vi "Denkovi_USB_4_8_RelayDemo.vi"() -> ()   [LabVIEW 2018]
panel:
  out "FT_Status":u32(ring) items=["FT_OK", "FT_INVALID_HANDLE", "FT_DEVICE_NOT_FOUND", "FT_DEVICE_NOT_OPENED", "FT_IO_ERROR", "FT_INSUFFICIENT_RESOURCES", "FT_INVALID_PARAMETER", "FT_INVALID_BAUD_RATE", "FT_DEVICE_NOT_OPENED_FOR_ERASE", "FT_DEVICE_NOT_OPENED_FOR_WRITE", "FT_FAILED_TO_WRITE_DEVICE", "FT_EEPROM_READ_FAILED", "FT_EEPROM_WRITE_FAILED", "FT_EEPROM_ERASE_FAILED", "FT_EEPROM_NOT_PRESENT", "FT_EEPROM_NOT_PROGRAMMED", "FT_INVALID_ARGS", "FT_NOT_SUPPORTED", "FT_OTHER_ERROR"]
  out "Device Description":string
  out "Pin States":T1
  in  "ALL ON/OFF":bool
  in  "DO7":bool
  in  "DO6":bool
  in  "DO5":bool
  in  "DO4":bool
  in  "DO3":bool
  in  "DO2":bool
  in  "DO1":bool
  in  "DO0":bool
  in  "Device Index":u32
  # "LabView demo example for USB 4/8 Relay Board by Denkovi\nDemonstrates how to read and write USB relay board I/O lines (relays). Uses the FTDI D2XX functions."
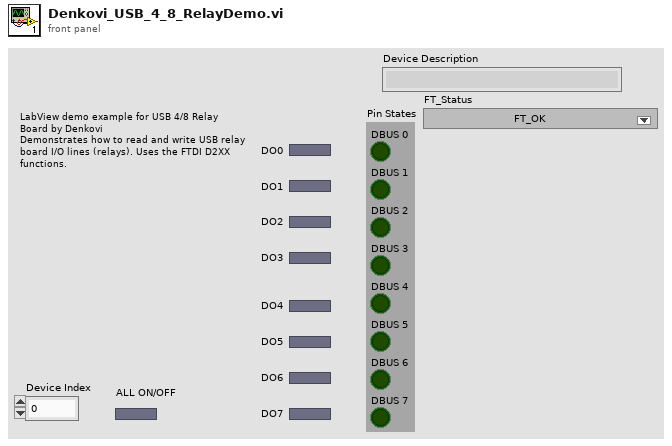
[diagram p1: front panel]
types:
  T1 = cluster{"DBUS 0":bool, "DBUS 1":bool, "DBUS 2":bool, "DBUS 3":bool, "DBUS 4":bool, "DBUS 5":bool, "DBUS 6":bool, "DBUS 7":bool}
  T2 = cluster{"Boolean array[0]":bool, "Boolean array[1]":bool, "Boolean array[2]":bool, "Boolean array[3]":bool, "Boolean array[4]":bool, "Boolean array[5]":bool, "Boolean array[6]":bool, "Boolean array[7]":bool}
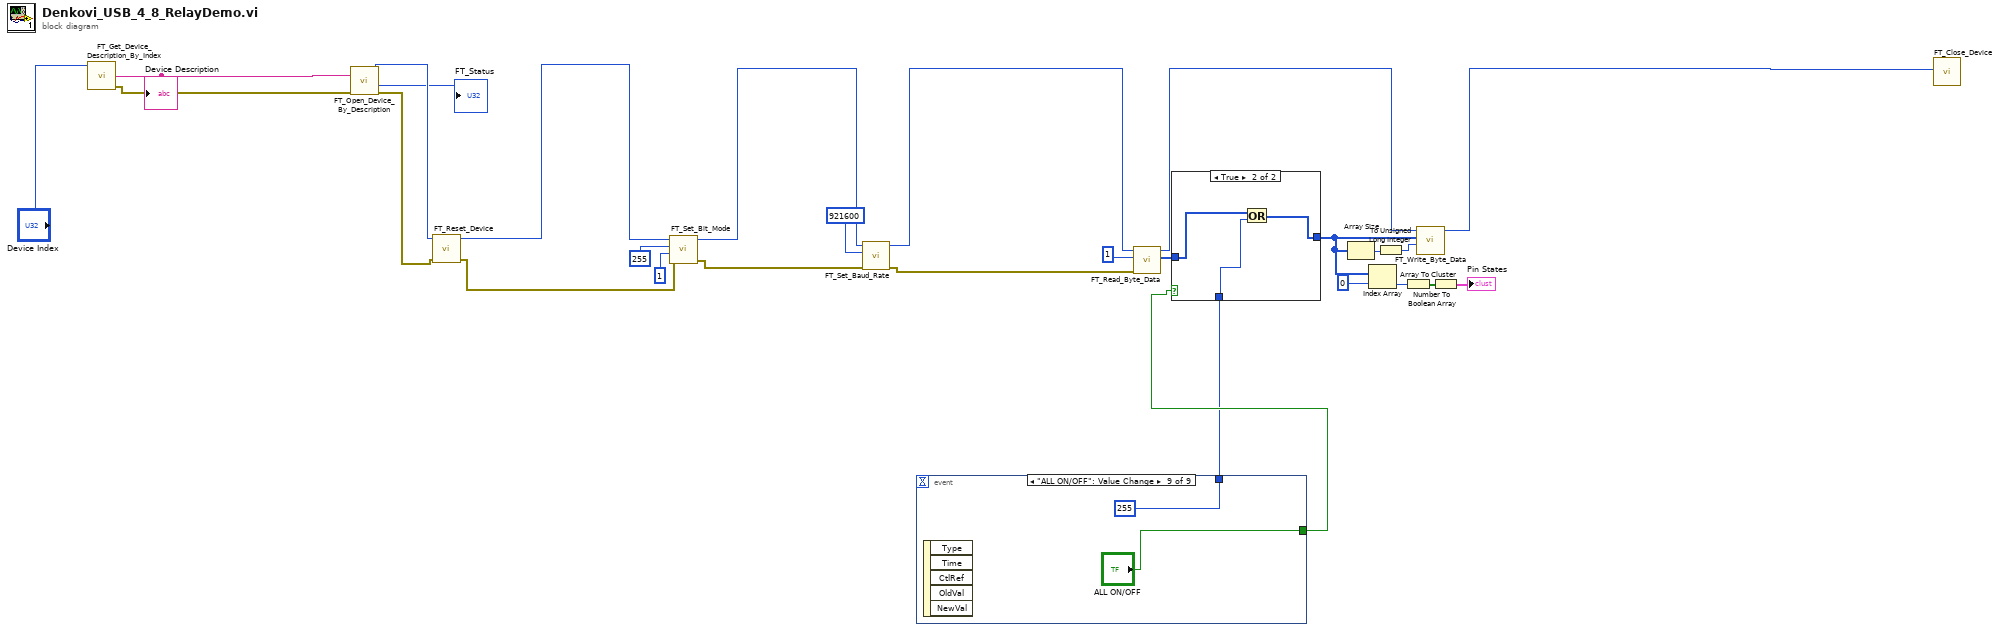
[diagram p0: block diagram]
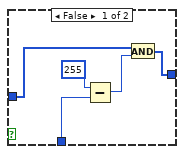
[diagram p2: hidden frame]
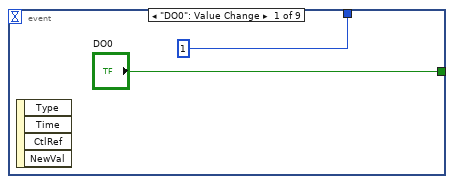
[diagram p3: hidden frame]
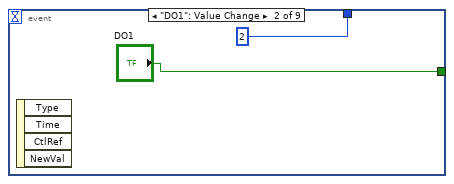
[diagram p4: hidden frame]
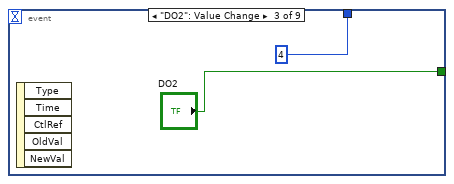
[diagram p5: hidden frame]
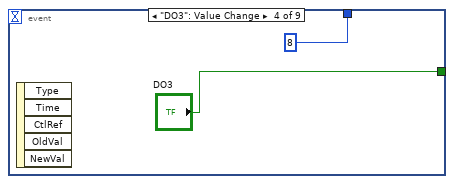
[diagram p6: hidden frame]
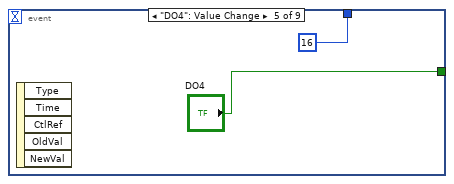
[diagram p7: hidden frame]
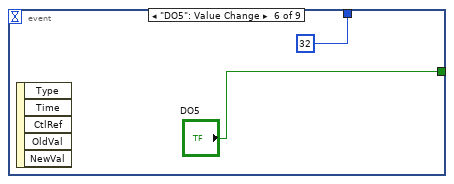
[diagram p8: hidden frame]
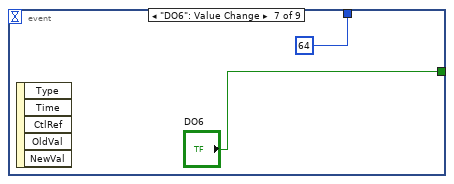
[diagram p9: hidden frame]
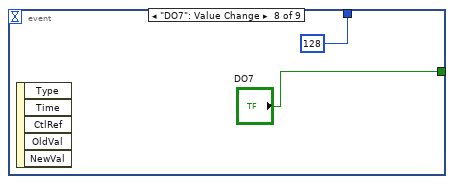
[diagram p10: hidden frame]
diagram:
  n1 = call "FT_Get_Device_Description_By_Index.vi"("Device Index"="Device Index") -> ("error out"=w24:errorcluster, "Device Description"=w28:string)  [unwired: 8 in, 1 out]
  "Device Description" <- w28
  n2 = call "FT_Open_Device_By_Description.vi"("error in (no error)"=w24, "Device Description"=w28) -> ("error out"=w5:errorcluster, "FT_Status"=→"FT_Status":u32, "Handle"=w10:u32)  [unwired: 7 in]
  n3 = call "FT_Reset_Device.vi"("error in (no error)"=w5, "Handle In"=w10) -> ("error out"=w4:errorcluster, "Handle Out"=w9:u32)  [unwired: 7 in, 1 out]
  n4 = call "FT_Set_Bit_Mode.vi"("error in (no error)"=w4, "Bit Mode"=1, "Bit Mode Mask"=255, "Handle In"=w9) -> ("error out"=w3:errorcluster, "Handle Out"=w8:u32)  [unwired: 5 in, 1 out]
  n5 = call "FT_Set_Baud_Rate.vi"("error in (no error)"=w3, "Baud Rate"=921600, "Handle  In"=w8) -> ("error out"=w2:errorcluster, "Handle Out"=w7:u32)  [unwired: 6 in, 1 out]
  n6 = event shown="[8] \"ALL ON/OFF\": Value Change" {
    selector: _ -> [_ _ _ _ _ _ _ _ _]
    dyn-events: _ -> [_ _ _ _ _ _ _ _ _]
    timeout: _ -> [_ _ _ _ _ _ _ _ _]
    tunnel: ["DO0" "DO1" "DO2" "DO3" "DO4" "DO5" "DO6" "DO7" "ALL ON/OFF"] -> w26
    tunnel: [1 2 4 8 16 32 64 128 255] -> w25
    event "DO0": Value Change {
      n7 = event-data() -> ()  [unwired: 1 in, 4 out]
    }
    event "DO1": Value Change {
      n8 = event-data() -> ()  [unwired: 1 in, 4 out]
    }
    event "DO2": Value Change {
      n9 = event-data() -> ()  [unwired: 1 in, 5 out]
    }
    event "DO3": Value Change {
      n10 = event-data() -> ()  [unwired: 1 in, 5 out]
    }
    event "DO4": Value Change {
      n11 = event-data() -> ()  [unwired: 1 in, 5 out]
    }
    event "DO5": Value Change {
      n12 = event-data() -> ()  [unwired: 1 in, 5 out]
    }
    event "DO6": Value Change {
      n13 = event-data() -> ()  [unwired: 1 in, 5 out]
    }
    event "DO7": Value Change {
      n14 = event-data() -> ()  [unwired: 1 in, 5 out]
    }
    event "ALL ON/OFF": Value Change {
      n15 = event-data() -> ()  [unwired: 1 in, 5 out]
    }
  }
  n16 = call "FT_Read_Byte_Data.vi"("error in (no error)"=w2, "Bytes To Read"=1, "Handle In"=w7) -> ("Read Data"=w18:u8[], "Handle Out"=w6:u32)  [unwired: 4 in, 3 out]
  n17 = case shown="True" w26 {
    tunnel: [w47 w52] -> w14
    tunnel: w18 -> [w49 w54]
    tunnel: w25 -> [w48 w53]
    frame False {
      n18 = Subtract(x=255, y=w48) -> (x-y=w51:i32)
      n19 = And(x=w49, y=w51) -> (x .and. y?=w47:i32[])
    }
    frame True {
      n20 = Or(x=w54, y=w53) -> (x .or. y?=w52:i32[])
    }
  }
  n21 = Array Size(array=w14) -> (size(s)=w21:i32)
  n22 = Index Array(array=w14, index=0) -> (element=w15:i32)
  n23 = To Unsigned Long Integer(number=w21) -> (unsigned 32bit integer=w22:u32)
  n24 = Number To Boolean Array(number=w15) -> (Boolean array=w16:bool[])
  n25 = call "FT_Write_Byte_Data.vi"("Bytes To Write"=w22, "Buffer"=w14, "Handle"=w6) -> ("Handle Out"=w27:u32)  [unwired: 5 in, 3 out]
  n26 = Array To Cluster(array=w16) -> (cluster=→"Pin States":T2)
  n27 = call "FT_Close_Device.vi"("Handle In"=w27) -> ()  [unwired: 8 in, 3 out]
